vi "Convert to Pump Interface State.vi"(8 "error in (no error)":errorcluster, 11 "Instrument State in":T2) -> (0 "error out":errorcluster, 3 "Instrument State out":variant)   [LabVIEW 2020, in "ChromTech Next Gen Compensator Pump.lvlib" / "Remote Connection Manager.lvlib"]
doc: "Converts the internal instrument state cluster into the remote instrument state representation."
uses:
  Remote Connection Manager.lvlib
  Instrument Manager/Instrument State.ctl
  Typedefs/Pump Controller State.ctl
  ChromTech Next Gen Compensator Pump.lvlib
  Instrument Manager/Instrument Manager.lvlib
panel:
  out "Pump Controller State":T1
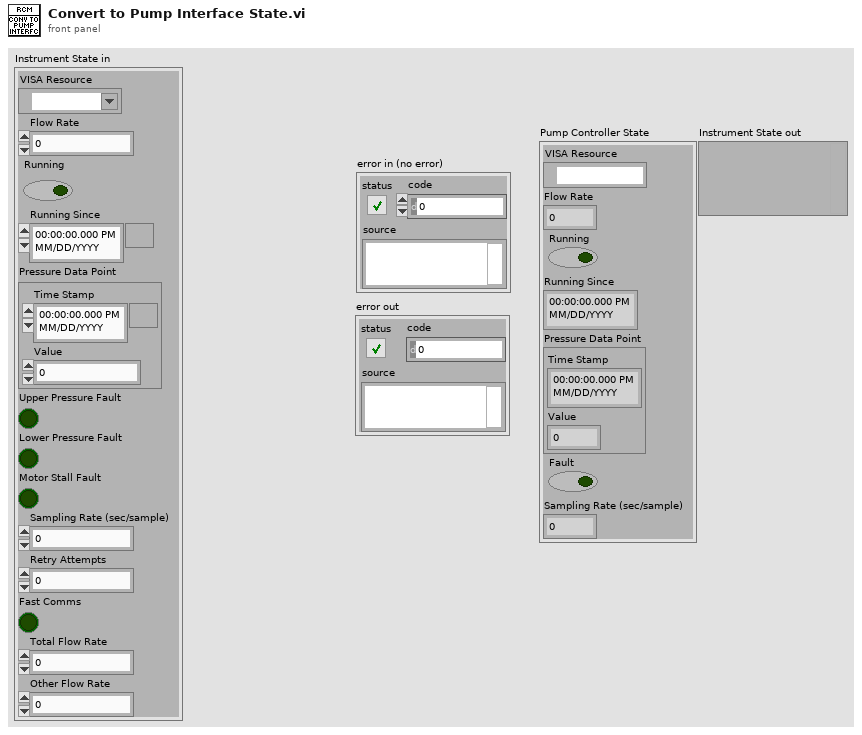
[diagram p1: front panel]
types:
  T1 = typedef "ChromTech Next Gen Compensator Pump.lvlib/Pump Controller State.ctl" = cluster{"VISA Resource":refnum<visa-resource-name>, "Flow Rate":dbl, "Running":bool, "Running Since":timestamp, "Pressure Data Point":cluster{"Time Stamp":timestamp, "Value":dbl}, "Fault":bool, "Sampling Rate (sec/sample)":dbl}
  T2 = typedef "ChromTech Next Gen Compensator Pump.lvlib/Instrument Manager.lvlib/Instrument State.ctl" = cluster{"VISA Resource":refnum<visa-resource-name>, "Flow Rate":dbl, "Running":bool, "Running Since":timestamp, "Pressure Data Point":cluster{"Time Stamp":timestamp, "Value":dbl}, "Upper Pressure Fault":bool, "Lower Pressure Fault":bool, "Motor Stall Fault":bool, "Sampling Rate (sec/sample)":dbl, "Retry Attempts":i32, "Fast Comms":bool, "Total Flow Rate":dbl, "Other Flow Rate":dbl}
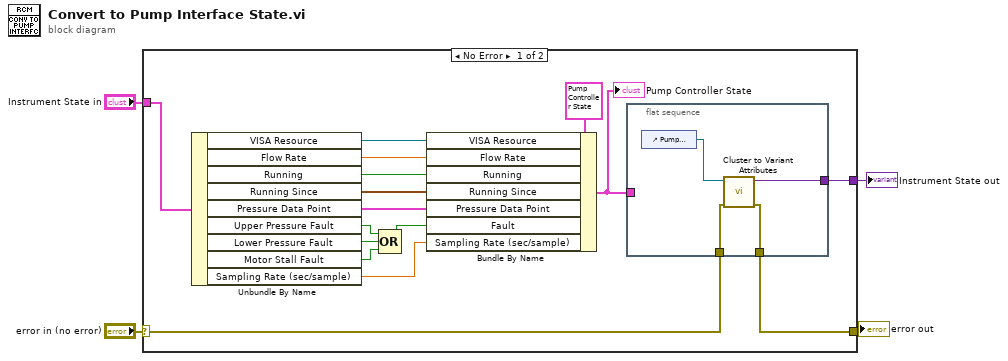
[diagram p0: block diagram]
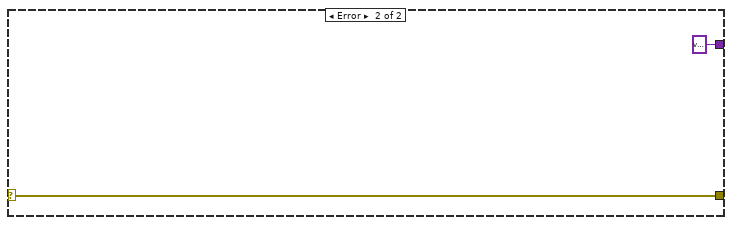
[diagram p2: hidden frame]
diagram:
  n1 = case shown="No Error" "error in (no error)" {
    selector: "error in (no error)" -> [w7 w26]
    tunnel: "Instrument State in" -> [w20 _]
    tunnel: [w6 w26] -> w2
    tunnel: [w8 variant ("Variant out")] -> w1
    frame No Error {
      n2 = Unbundle By Name(w20) -> ("VISA Resource"=w18:refnum<visa-resource-name>, "Flow Rate"=w17:dbl, "Running"=w16:bool, "Running Since"=w15:timestamp, "Pressure Data Point"=w14:cluster{"Time Stamp":timestamp, "Value":dbl}, "Upper Pressure Fault"=w13:bool, "Lower Pressure Fault"=w12:bool, "Motor Stall Fault"=w11:bool, "Sampling Rate (sec/sample)"=w9:dbl)
      n3 = Compound Arithmetic op=OR(w13, w12, w11) -> (w10:bool)
      n4 = Bundle By Name(cluster=T1 {"VISA Resource"="", "Flow Rate"=0.0, "Running"=FALSE, "Running Since"=timestamp(0 s since 1904-01-01), "Pressure Data Point"={"Time Stamp"=timestamp(0 s since 1904-01-01), "Value"=0.0}, "Fault"=FALSE, "Sampling Rate (sec/sample)"=0.0} ("Pump Controller State"), "VISA Resource"=w18, "Flow Rate"=w17, "Running"=w16, "Running Since"=w15, "Pressure Data Point"=w14, "Fault"=w10, "Sampling Rate (sec/sample)"=w9) -> (w5:T1)
      "Pump Controller State" <- w5
      n5 = flat-sequence {
        tunnel: [w23] -> w8
        tunnel: w7 -> [w22]
        tunnel: [w21] -> w6
        tunnel: w5 -> [_]
        frame #0 {
          n6 = control-ref of="Pump Controller State"() -> (w24:refnum<vi>)
          n7 = call "Cluster to Variant Attributes.vi"("error in (no error)"=w22, "Cluster in"=w24) -> ("error out"=w21:errorcluster, "Variant out"=w23:variant)  [unwired: 8 in]
        }
      }
    }
    frame Error {
    }
  }
  "error out" <- w2
  "Instrument State out" <- w1
